vi "6009analoginputdatalogging.vi"() -> ()   [LabVIEW 2012]
panel:
  in  "stop (F)":bool
  out "Waveform Graph 2":dynamicdata(graph)
  out "Waveform Graph":dynamicdata(graph)
  # "This example code assumes your Device name is Dev1.\n\nTo change this VI's settings to match your device name, go to the diagram of this VI, double-click on the DAQ Assistant and under \"Channel settings\" right-click on each channel and select \"Change Physical Channel\". Then choose the device name that matches your device."
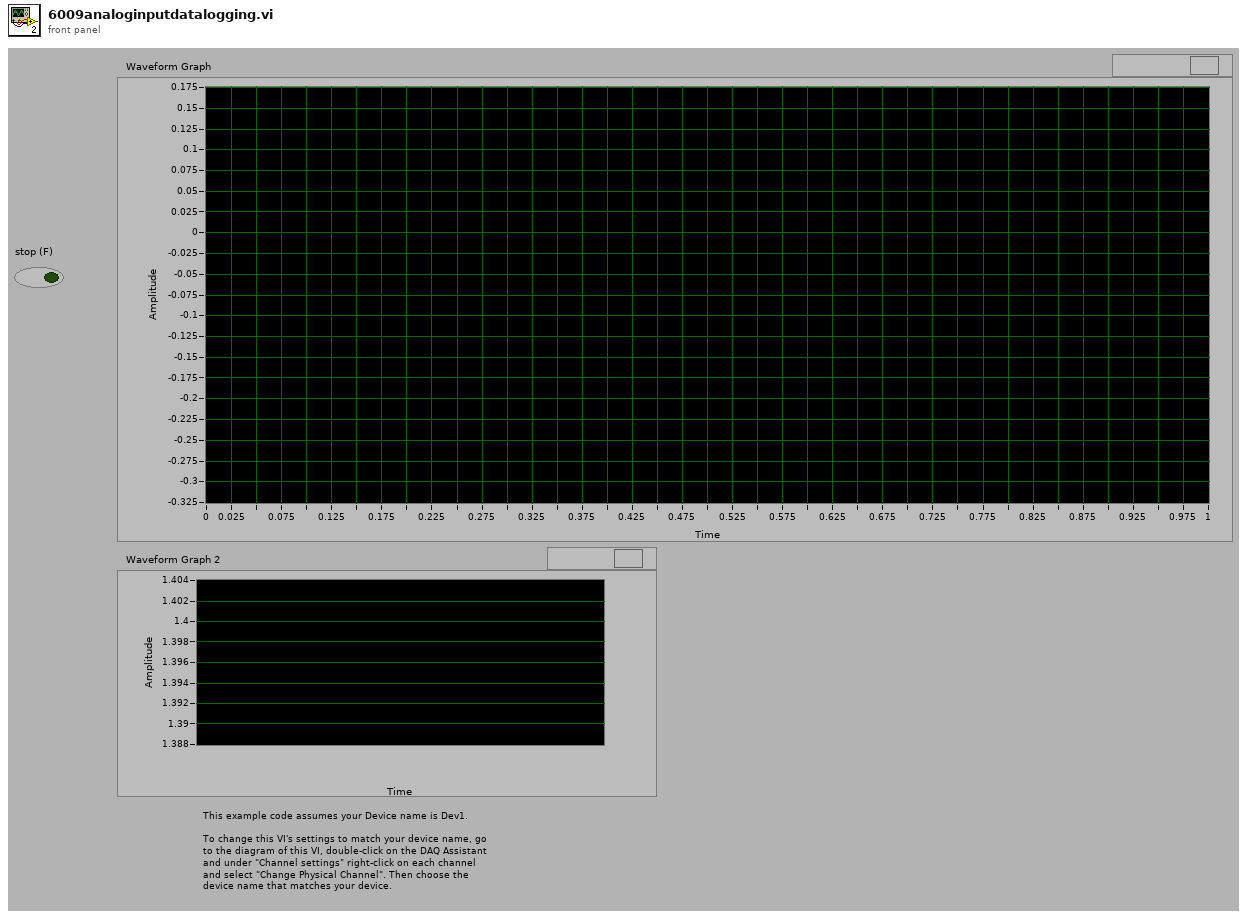
[diagram p1: front panel]
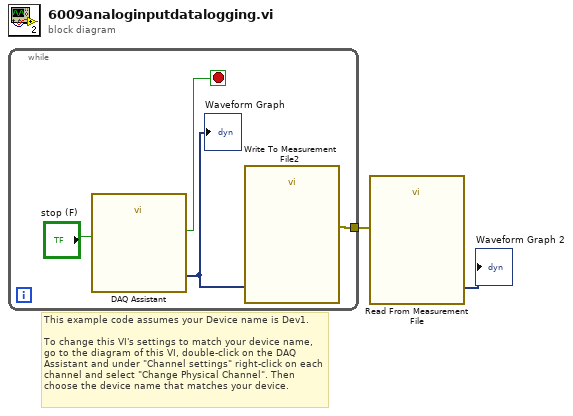
[diagram p0: block diagram]
diagram:
  # "This example code assumes your Device name is Dev1.\n\nTo change this VI's settings to match your device name, go to the diagram of this VI, double-click on the DAQ Assistant and under \"Channel settings\" right-click on each channel and select \"Change Physical Channel\". Then choose the device name that matches your device."
  n1 = while {
    tunnel: [w3] -> w1
    stop <- w5 stop-if-true
    n2 = call "DAQ Assistant"("stop (F)"="stop (F)") -> ("data"=w4:dynamicdata, "stopped"=w5:bool)  [unwired: 5 in, 12 out]
    "Waveform Graph" <- w4
    n3 = call "Write To Measurement File2"("Signals"=w4) -> ("error out"=w3:errorcluster)  [unwired: 16 in, 2 out]
  }
  n4 = call "Read From Measurement File"("error in (no error)"=w1) -> ("Signals"=→"Waveform Graph 2":dynamicdata)  [unwired: 3 in, 7 out]
